vi "Compare New Values.vi"(8 "error in (no error)":errorcluster, 10 "New Values":string[](array[string]), 11 "Selector in":refnum<class "Selector.lvclass">) -> (0 "error out":errorcluster, 2 "Unchanged ?":bool, 3 "Selector out":refnum<class "Selector.lvclass">)   [LabVIEW 2019, in "Selector.lvclass"]
uses:
  Selector.lvclass
  Selector.lvclass/Selector.ctl
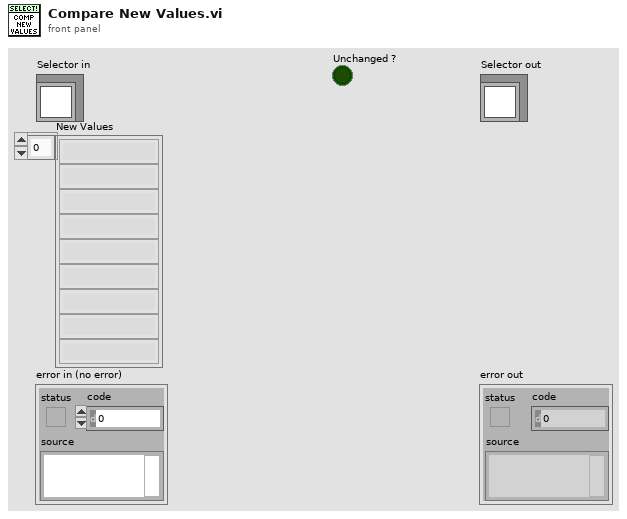
[diagram p1: front panel]
types:
  T1 = cluster{"Name":string, "Group":string, "Enabled":bool}[]
  T2 = cluster{"Name":string, "Group":string, "Enabled":bool}
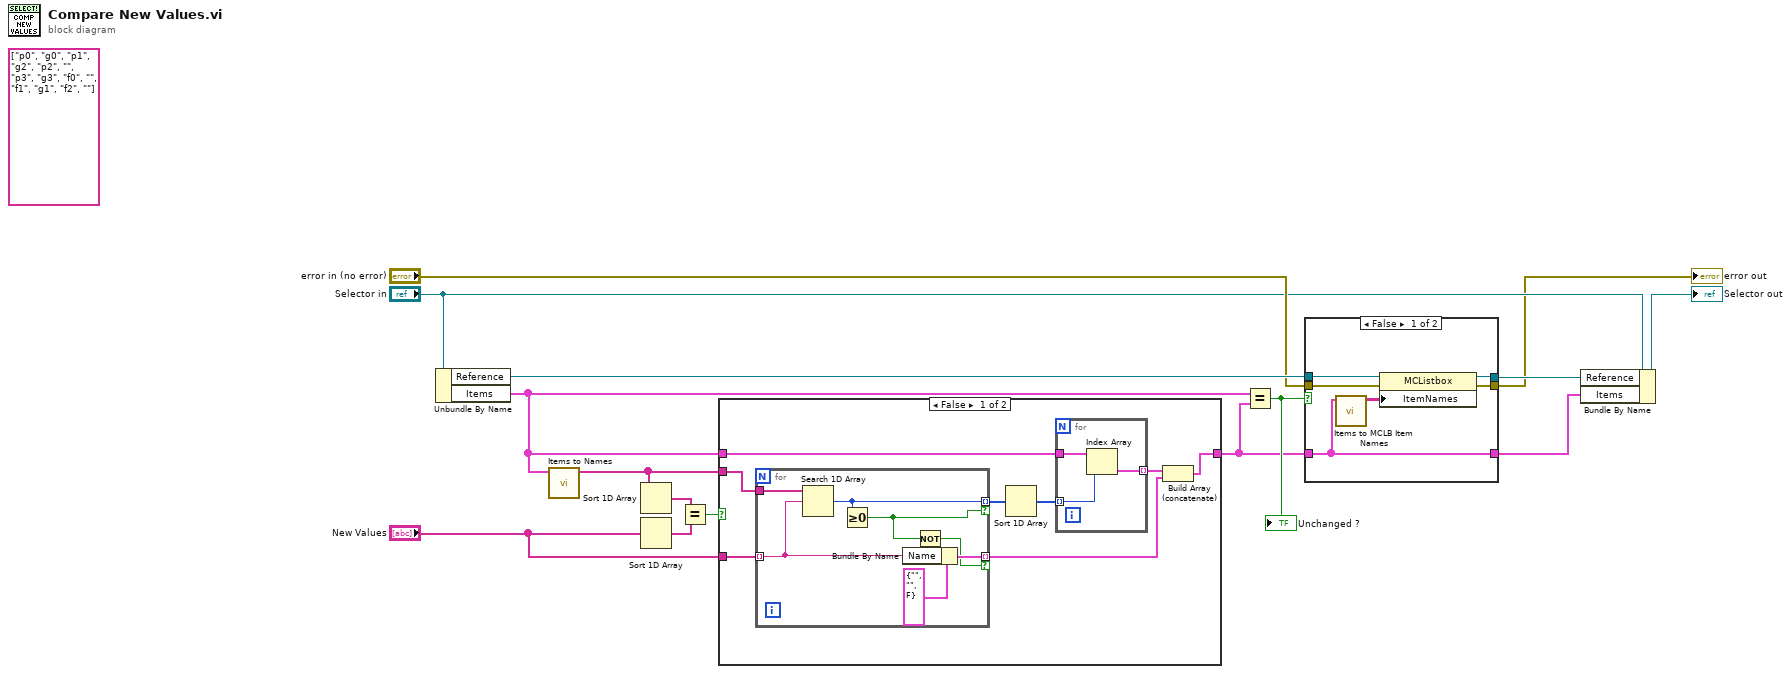
[diagram p0: block diagram]
diagram:
  (unwired) string[][] [["p0", "g0"], ["p1", "g2"], ["p2", ""], ["p3", "g3"], ["f0", ""], ["f1", "g1"], ["f2", ""]] ("Item Names")
  n1 = Unbundle By Name("Selector in") -> ("Reference"=w8:refnum<vi>, "Items"=w9:T1)
  n2 = call "Items to Names.vi"("Items"=w9) -> ("Names"=w12:string[])  [unwired: 6 in]
  n3 = Sort 1D Array(array=w12) -> (sorted array=w15:string[])
  n4 = Sort 1D Array(array="New Values") -> (sorted array=w14:string[])
  n5 = Equal?(x=w15, y=w14) -> (x = y?=w13:bool)
  n6 = case shown="False" w13 {
    tunnel: w9 -> [w20 w34]
    tunnel: w12 -> [w23 _]
    tunnel: "New Values" -> [w22 _]
    tunnel: [w16 w34] -> w7
    frame False {
      n7 = for {
        tunnel: w23 -> [w33]
        tunnel: w22 -> [w29] mode=indexing
        tunnel: [w31] -> w21 mode=indexing if=w27
        tunnel: [w30] -> w17 mode=indexing if=w28
        n8 = Search 1D Array(1D array=w33, element=w29) -> (index of element=w31:i32)  [unwired: 1 in]
        n9 = Greater Or Equal To 0?(x=w31) -> (x >= 0?=w27:bool)
        n10 = Bundle By Name(cluster=T2 {"Name"="", "Group"="", "Enabled"=FALSE} ("Item"), "Name"=w29) -> (w30:T2)
        n11 = Not(x=w27) -> (.not. x?=w28:bool)
      }
      n12 = Sort 1D Array(array=w21) -> (sorted array=w19:i32[])
      n13 = for {
        tunnel: w20 -> [w26]
        tunnel: w19 -> [w25] mode=indexing
        tunnel: [w24] -> w18 mode=indexing
        n14 = Index Array(array=w26, index=w25) -> (element=w24:T2)
      }
      n15 = Build Array (concatenate)(w18, w17) -> (w16:T1)
    }
    frame True {
    }
  }
  n16 = Equal?(x=w9, y=w7) -> (x = y?=w10:bool)
  "Unchanged ?" <- w10
  n17 = case shown="False" w10 {
    tunnel: w8 -> [w40 w42]
    tunnel: w7 -> [w35 w43]
    tunnel: [w38 w42] -> w6
    tunnel: [w37 w41] -> w1
    tunnel: "error in (no error)" -> [w36 w41]
    tunnel: [w35 w43] -> w5
    frame False {
      n18 = call "Items to MCLB Item Names.vi"("Items"=w35) -> ("Item Names"=w39:string[][])  [unwired: 6 in]
      n19 = property class="MCListbox"(reference=w40, error in=w36, "ItemNames"=w39) -> (reference out=w38:refnum<vi>, error out=w37:errorcluster)
    }
    frame True {
    }
  }
  "error out" <- w1
  n20 = Bundle By Name(cluster="Selector in", "Reference"=w6, "Items"=w5) -> (→"Selector out":refnum<class "Selector.lvclass">)
